vi "Merge AO Settings to Generator.vi"(8 "error in (no error)":errorcluster, 11 "Instrument.DAQ in":refnum<class "Instrument.DAQ.lvclass">) -> (0 "error out":errorcluster, 2 "AO Channels":T1, 3 "Instrument.DAQ out":refnum<class "Instrument.DAQ.lvclass">)   [LabVIEW 2019, in "Instrument.Lockin.lvlib" / "Instrument.DAQ.lvclass"]
uses:
  Instrument.DAQ.lvclass
  Generator/typedefs/AO.Channel--Cluster--Array.ctl
  Generator/typedefs/AO.Channel--Cluster.ctl
  Generator/typedefs/AO.Channel.Function--Enum.ctl
  Instrument.DAQ.lvclass/Instrument.DAQ.ctl
  Typedefs/AO.Channel--Cluster.ctl
  Typedefs/AO.Channel.Function--Enum.ctl
  Generator/Generator.lvclass
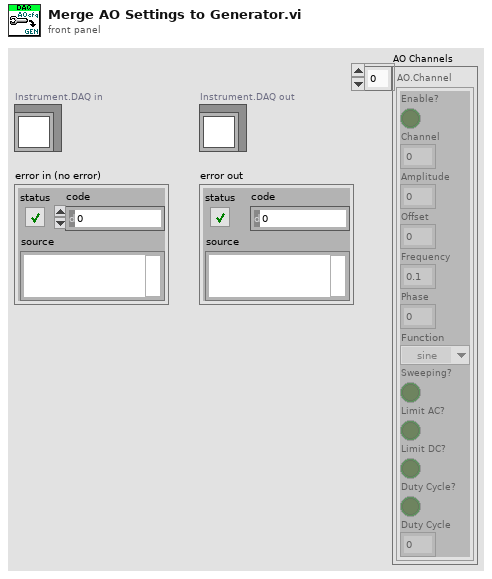
[diagram p1: front panel]
types:
  T1 = typedef "Generator.lvclass/AO.Channel--Cluster--Array.ctl" = T2[]
  T2 = typedef "Generator.lvclass/AO.Channel--Cluster.ctl" = cluster{"Enable?":bool, "Channel":i32, "Amplitude":dbl, "Offset":dbl, "Frequency":dbl, "Phase":dbl, "Function":T3, "Sweeping?":bool, "Limit AC?":bool, "Limit DC?":bool, "Duty Cycle?":bool, "Duty Cycle":dbl}
  T3 = typedef "Generator.lvclass/AO.Channel.Function--Enum.ctl" = enum16{"sine", "square", "triangle", "saw"}
  T4 = typedef "Instrument.Lockin.lvlib/Instrument.DAQ.lvclass/AO.Channel--Cluster.ctl" = cluster{"Enable?":bool, "Channel":i32, "Amplitude":dbl, "Offset":dbl, "Frequency":dbl, "Phase":dbl, "Function":T5, "Sweeping?":bool, "Limit AC":bool, "Limit DC?":bool, "Duty Cycle":bool}
  T5 = typedef "Instrument.Lockin.lvlib/Instrument.DAQ.lvclass/AO.Channel.Function--Enum.ctl" = enum16{"sine", "square", "triangle", "saw"}
  T6 = typedef "Instrument.Lockin.lvlib/Instrument.DAQ.lvclass/AO.Channel--Cluster--Array.ctl" = T4[]
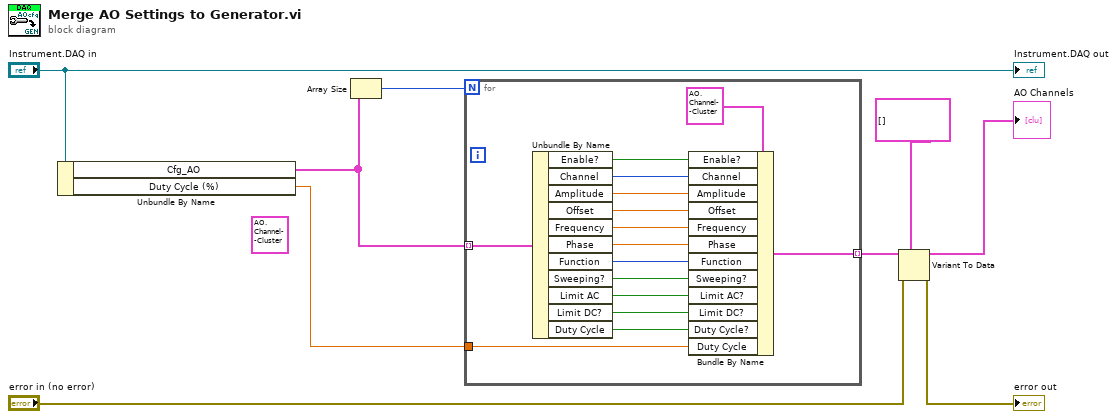
[diagram p0: block diagram]
diagram:
  (unwired) T4 {"Enable?"=TRUE, "Channel"=0, "Amplitude"=0.0, "Offset"=0.0, "Frequency"=10.0, "Phase"=0.0, "Function"=enum."sine", "Sweeping?"=TRUE, "Limit AC"=TRUE, "Limit DC?"=TRUE, "Duty Cycle"=TRUE} ("input cluster")
  n1 = Unbundle By Name("Instrument.DAQ in") -> ("Cfg_AO"=w6:T6, "Duty Cycle (%)"=w9:dbl)
  n2 = Array Size(array=w6) -> (size(s)=w7:i32)
  n3 = for {
    N: w7 -> [_]
    tunnel: w6 -> [w24] mode=indexing
    tunnel: w9 -> [w23]
    tunnel: [w11] -> w5 mode=indexing
    n4 = Unbundle By Name(w24) -> ("Enable?"=w22:bool, "Channel"=w13:i32, "Amplitude"=w14:dbl, "Offset"=w15:dbl, "Frequency"=w16:dbl, "Phase"=w17:dbl, "Function"=w12:T5, "Sweeping?"=w18:bool, "Limit AC"=w19:bool, "Limit DC?"=w20:bool, "Duty Cycle"=w21:bool)
    n5 = Bundle By Name(cluster=T2 {"Enable?"=FALSE, "Channel"=0, "Amplitude"=0.0, "Offset"=0.0, "Frequency"=0.1, "Phase"=0.0, "Function"=enum."sine", "Sweeping?"=FALSE, "Limit AC?"=FALSE, "Limit DC?"=FALSE, "Duty Cycle?"=FALSE, "Duty Cycle"=0.0} ("AO.Channel"), "Enable?"=w22, "Channel"=w13, "Amplitude"=w14, "Offset"=w15, "Frequency"=w16, "Phase"=w17, "Function"=w12, "Sweeping?"=w18, "Limit AC?"=w19, "Limit DC?"=w20, "Duty Cycle?"=w21, "Duty Cycle"=w23) -> (w11:T2)
  }
  n6 = Variant To Data(error in="error in (no error)", type=T1 [] ("AO Channels"), Variant=w5) -> (data=→"AO Channels":T1, error out=→"error out":errorcluster)
  "Instrument.DAQ out" <- "Instrument.DAQ in"
